vi "binary_approx_sumOfFrequencies.vi"(6 "frequency":dbl, 9 "signal type":enum16{"Sine", "Square", "Sawtooth", "Random"}(ring), 10 "offset":dbl, 11 "amplitude":dbl) -> (3 "Numeric":dbl)   [LabVIEW 2020]
uses:
  sumOfFrequencies.vi
  <vilib>/Simulation/Implementation/Shared/SIMSCR Execution Mode.ctl
  <vilib>/Simulation/Scripting/Companion Diagram/SimConfigNode/SimParams.ctl
  <vilib>/Simulation/Scripting/Companion Diagram/SimConfigNode/_simSolvers.ctl
  <vilib>/Simulation/Param Hierarchy/Typedefs/SIMPH Param Control Actions.ctl
  <vilib>/Simulation/Implementation/Shared/NILVSim_ParamChanged.vi
  <vilib>/Simulation/Implementation/Shared/NILVSIM_BeginStep.vi
  <vilib>/Simulation/Implementation/Shared/NILVSim_Manager.vi
  <vilib>/Utility/error.llb/Clear Errors.vi
  <vilib>/Simulation/Implementation/Shared/NILVSim_FinalizeModel.vi
  <vilib>/Simulation/Implementation/Shared/SIM Unbundle Sim Info.vi
  <vilib>/Simulation/Implementation/Shared/NILVSim_Initialize.vi
  <vilib>/Simulation/Utility/Implementation/NILVSim Get Time and IsAcceptedStep.vi
  <vilib>/Simulation/Implementation/Shared/NILVSim_GetModelError.vi
  <vilib>/Simulation/Implementation/Shared/SIM SimErrorHandler.vi
  <vilib>/Simulation/Implementation/Shared/SIMSH Read Queue.vi
  <vilib>/Simulation/Implementation/Shared/SIM Bundle Sim Info.vi
  <vilib>/Simulation/Scripting/Companion Diagram/SimConfigNode/SimDog.xnode
  <vilib>/Simulation/Implementation/XNodeFramework/SimXNode/SimX.xnode
  <vilib>/Simulation/Implementation/Shared/NI_SIM_Implementation.lvlib
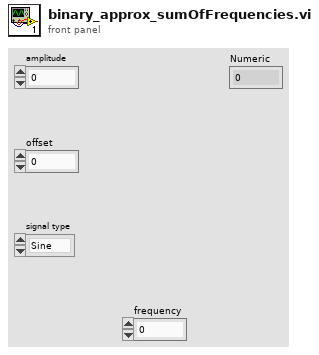
[diagram p1: front panel]
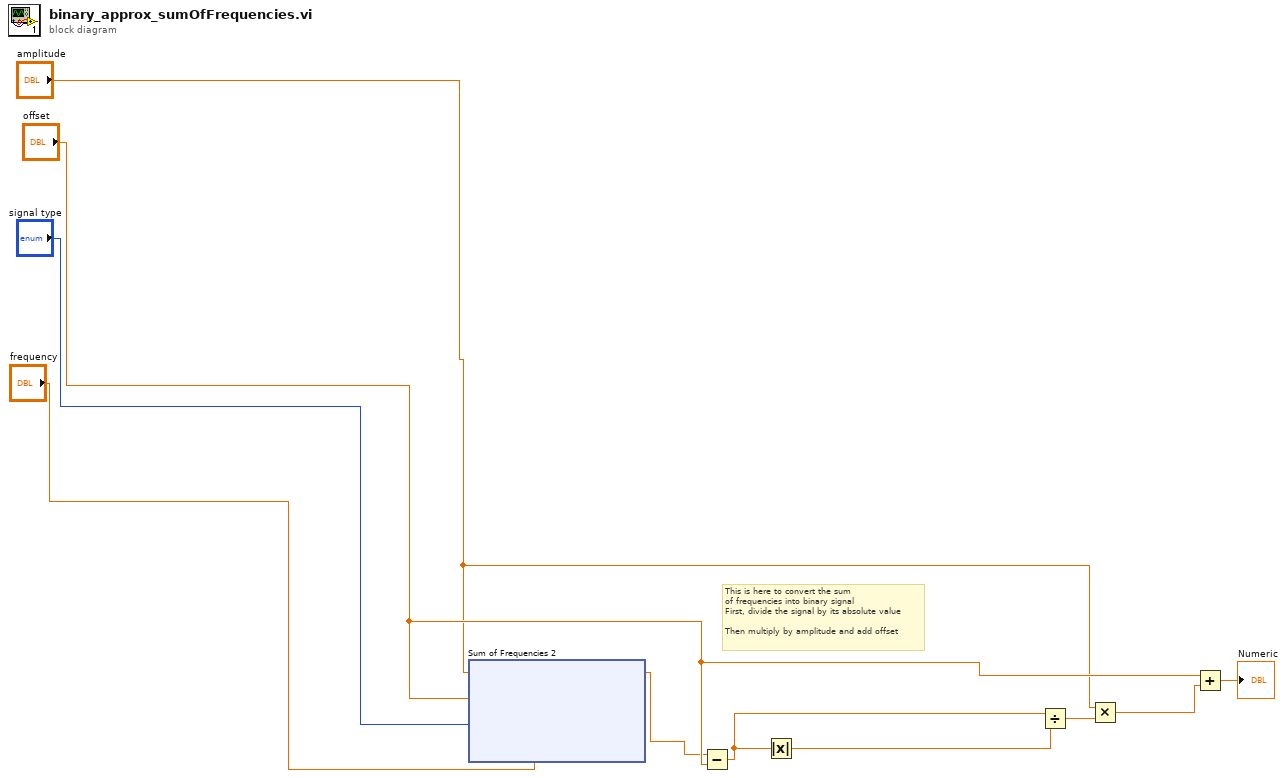
[diagram p0: block diagram]
diagram:
  # "This is here to convert the sum\nof frequencies into binary signal\nFirst, divide the signal by its absolute value\n\nThen multiply by amplitude and add offset"
  n1 = xnode "Sum of Frequencies 2"("frequency"="frequency", "signal type"="signal type", "offset"="offset", "amplitude"="amplitude") -> ("Numeric"=w4:dbl)  [unwired: 7 out]
  n2 = Subtract(x=w4, y="offset") -> (x-y=w5:dbl)
  n3 = Absolute Value(x=w5) -> (abs(x)=w3:dbl)
  n4 = Divide(x=w5, y=w3) -> (x/y=w6:dbl)
  n5 = Multiply(x="amplitude", y=w6) -> (x*y=w9:dbl)
  n6 = Add(x="offset", y=w9) -> (x+y=→"Numeric":dbl)
